vi "DSF.Engine.Sequencer.Create.vi"(8 "error in (no error)":errorcluster, 10 "Framework Configuration":refnum<class "DSF.Shared.Configuration.Framework.lvclass">, 11 "Sequencer type-specifier":refnum<class "DSF.Engine.Sequencer.lvclass">) -> (0 "error out":errorcluster, 3 "Sequencer":refnum<class "DSF.Engine.Sequencer.lvclass">)   [LabVIEW 2016, in "DSF.Engine.lvlib" / "DSF.Engine.Sequencer.lvclass"]
uses:
  DSF.Engine.Sequencer.lvclass
  Shared/Classes/Transfer Group/DSF.Shared.Configuration.Transfer Group.lvclass
  Shared/Classes/Transfer/DSF.Shared.Configuration.Transfer.lvclass
  Shared/Classes/Framework/DSF.Shared.Configuration.Framework.lvclass
  Timing/DSF.Engine.Timing.lvclass
  Plugin/DSF.Engine.Runtime.Plugin.lvclass
panel:
  in  "Plugin Runtimes":refnum<class "DSF.Engine.Runtime.Plugin.lvclass">[](array[class])
  in  "Timing":refnum<class "DSF.Engine.Timing.lvclass">
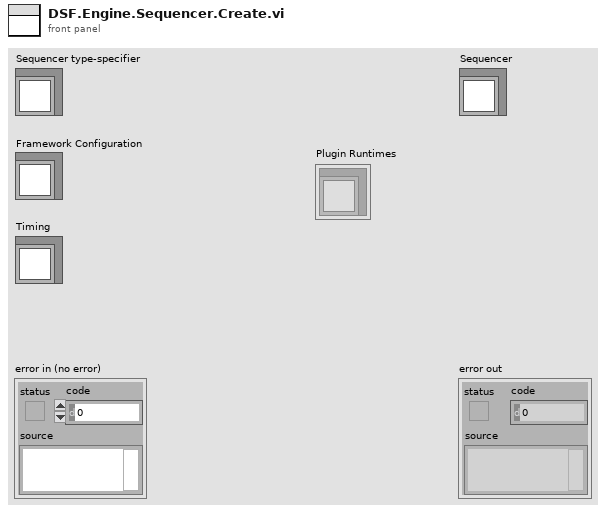
[diagram p1: front panel]
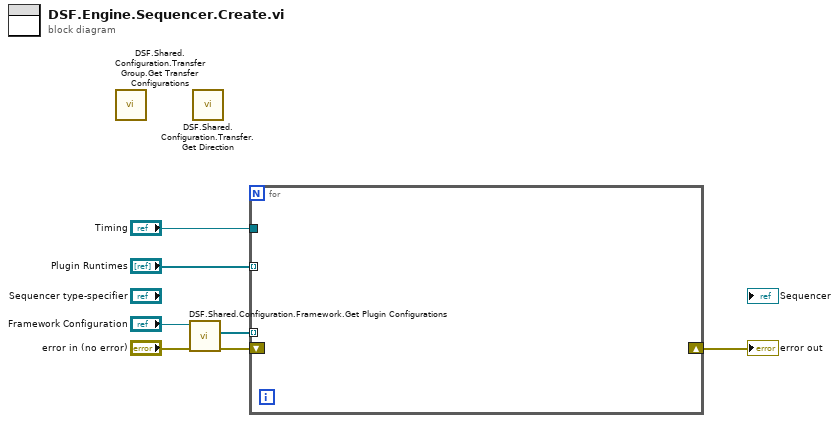
[diagram p0: block diagram]
diagram:
  n1 = call "DSF.Shared.Configuration.Transfer Group.Get Transfer Configurations.vi"() -> ()  [unwired: 9 in, 3 out]
  n2 = call "DSF.Shared.Configuration.Framework.Get Plugin Configurations.vi"("error in (no error)"="error in (no error)", "Framework Configuration in"="Framework Configuration") -> ("error out"=w5:errorcluster, "Plugin Configurations"=w3:refnum<class "DSF.Shared.Configuration.Plugin.lvclass">[])  [unwired: 7 in, 1 out]
  n3 = call "DSF.Shared.Configuration.Transfer.Get Direction.vi"() -> ()  [unwired: 9 in, 3 out]
  n4 = for {
    shift-right: [_] -> w4
    shift-left: w5 -> [_]
    tunnel: w3 -> [_] mode=indexing
    tunnel: "Plugin Runtimes" -> [_] mode=indexing
    tunnel: "Timing" -> [_]
  }
  "error out" <- w4
